vi "BitPacking.vi"(10 "Bits":u8=12, 11 "Array":u16[](array[numeric])=[4656, 17760, 30864] format="%04x") -> (2 "Pixels":i32, 3 "ByteArray":u8[](array[numeric]) format="%02x", 5 "Bytes":u32, 7 "Pixel":u32)   [LabVIEW 2011]
panel:
  # "größer out:15bytes; 15bit 8zu15, 8byte ginge in U64\ngrößter in:8Pixel; 1,3,5,7,9,11,13.15 bit 8zu x"
  # "no offset alyways msb!"
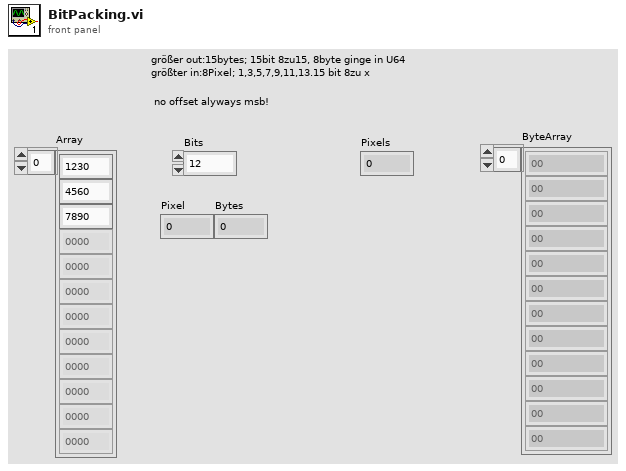
[diagram p1: front panel]
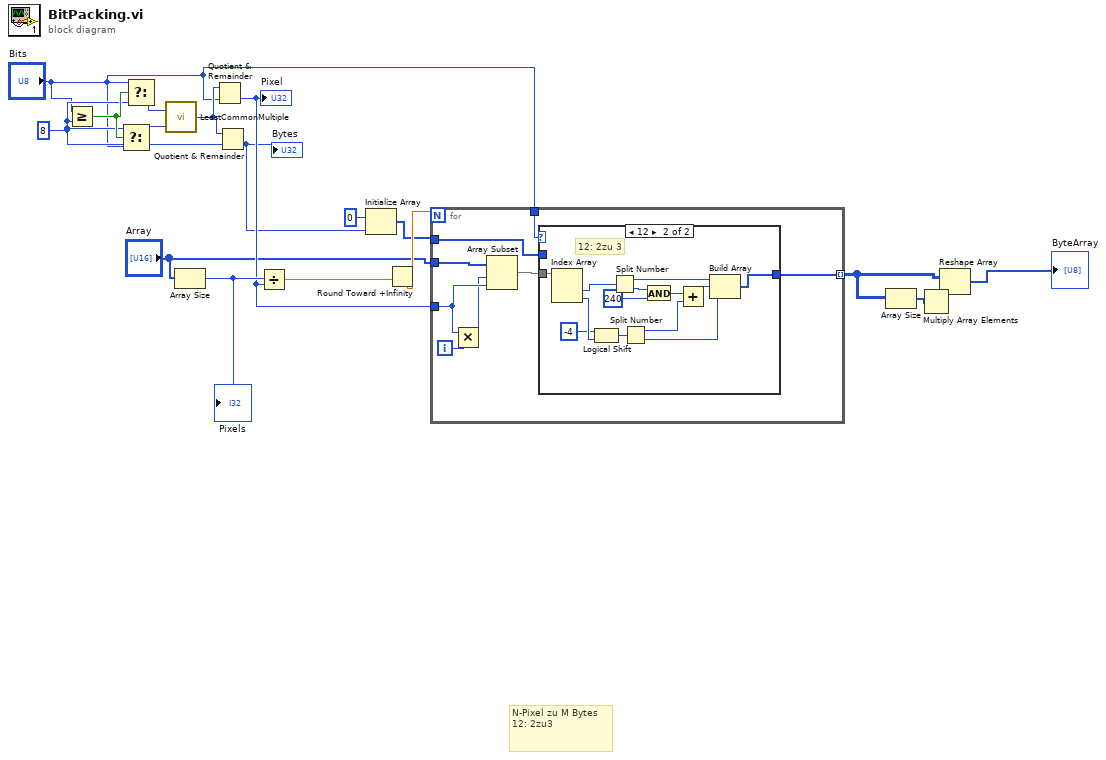
[diagram p0: block diagram]
diagram:
  w14 = u32 8 ("Numeric (larger)")
  # "N-Pixel zu M Bytes\n12: 2zu3"
  n1 = Greater Or Equal?(x="Bits", y=w14) -> (x >= y?=w16:bool)
  n2 = Select(t=w14, s=w16, f="Bits") -> (s? t:f=w17:u32)
  n3 = Select(t="Bits", s=w16, f=w14) -> (s? t:f=w18:u32)
  n4 = call "LeastCommonMultiple.vi"("Numeric (larger)"=w17, "Numeric"=w18) -> ("LCM"=w15:u32)
  n5 = Array Size(array="Array") -> (size(s)=w13:i32)
  "Pixels" <- w13
  n6 = Quotient & Remainder(x=w15, y="Bits") -> (floor(x/y)=w10:u32)  [unwired: 1 out]
  "Pixel" <- w10
  n7 = Quotient & Remainder(x=w15, y=w14) -> (floor(x/y)=w9:u32)  [unwired: 1 out]
  "Bytes" <- w9
  n8 = Divide(x=w13, y=w10) -> (x/y=w12:dbl)
  n9 = Initialize Array(u8 0 ("element"), w9) -> (w7:u8[])
  n10 = Round Toward +Infinity(x=w12) -> (ceil(x): smallest int >= x=w11:dbl)
  n11 = for {
    N: w11 -> [_]
    tunnel: "Array" -> [w26]
    tunnel: w10 -> [w24]
    tunnel: w7 -> [w19]
    tunnel: "Bits" -> [w21]
    tunnel: [w20] -> w4 mode=indexing
    i -> [w25]
    n12 = Multiply(x=w24, y=w25) -> (x*y=w23:u32)
    n13 = Array Subset(array=w26, index=w23, length=w24) -> (w22:u16[])
    n14 = case shown="12" w21 {
      tunnel: w22 -> [_ w40]
      tunnel: [w27 w32] -> w20
      tunnel: w19 -> [w27 _]
      frame 0, Default {
      }
      frame 12 {
        # "12: 2zu 3"
        n15 = Index Array(array=w40) -> (element #1=w39:u16, element #2=w38:u16)  [unwired: 2 in]
        n16 = Logical Shift(y=i8 -4, x=w38) -> (x << y=w37:u16)
        n17 = Split Number(x=w39) -> (hi(x)=w35:u8, lo(x)=w31:u8)
        n18 = Split Number(x=w37) -> (hi(x)=w28:u8, lo(x)=w33:u8)
        n19 = And(x=w31, y=u8 240) -> (x .and. y?=w29:u8)
        n20 = Add(x=w29, y=w28) -> (x+y=w34:u8)
        n21 = Build Array(w35, w34, w33) -> (w32:u8[])
      }
    }
  }
  n22 = Array Size(array=w4) -> (size(s)=w3:i32[])
  n23 = Multiply Array Elements(1:w3) -> (0:w2:i32)
  n24 = Reshape Array(w4, w2) -> (→"ByteArray":u8[])
